vi "8.8.vi"() -> ()   [LabVIEW 2017]
panel:
  out "XY Graph":cluster{i32[], dbl[]}(graph)
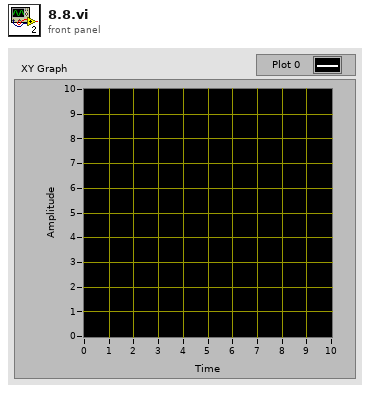
[diagram p1: front panel]
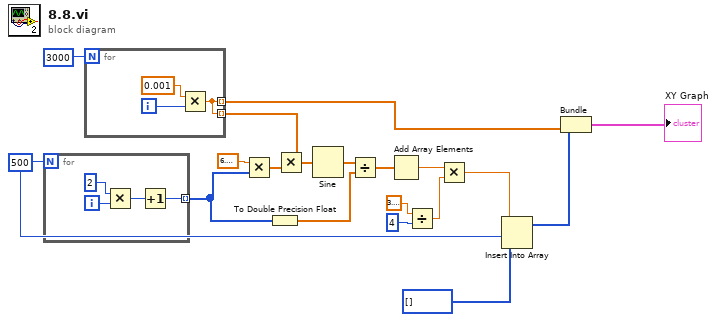
[diagram p0: block diagram]
diagram:
  w4 = 500
  n1 = for {
    N: w4 -> [_]
    tunnel: [w20] -> w2 mode=indexing
    i -> [w22]
    n2 = Multiply(x=2, y=w22) -> (x*y=w21:i32)
    n3 = Increment(x=w21) -> (x+1=w20:i32)
  }
  n4 = for {
    N: 3000 -> [_]
    tunnel: [w24] -> w17 mode=indexing
    tunnel: [w24] -> w8 mode=indexing
    i -> [w25]
    n5 = Multiply(x=0.001, y=w25) -> (x*y=w24:dbl)
  }
  n6 = Multiply(x=6.283185307179586, y=w2) -> (x*y=w16:dbl[])
  n7 = To Double Precision Float(number=w2) -> (double precision float=w1:dbl[])
  n8 = Multiply(x=w17, y=w16) -> (x*y=w15:dbl[])
  n9 = Sine(x=w15) -> (sin(x)=w14:dbl[])
  n10 = Divide(x=w14, y=w1) -> (x/y=w13:dbl[])
  n11 = Add Array Elements(numeric array=w13) -> (sum=w10:dbl)
  n12 = Divide(x=3.141592653589793, y=4) -> (x/y=w9:dbl)
  n13 = Multiply(x=w10, y=w9) -> (x*y=w6:dbl)
  n14 = Insert Into Array(array=i32[] [], index=w4, new element=w6) -> (w5:i32[])
  n15 = Bundle(w5, w8) -> (→"XY Graph":cluster{i32[], dbl[]})  [unwired: 1 in]
